vi "Picture to 4bit Picture.vi"() -> ()   [LabVIEW 2014]
uses:
  <userlib>/_OpenG.lib/file/file.llb/Strip Path Extension - Path__ogtk.vi
  <vilib>/Utility/error.llb/Error Cluster From Error Code.vi
  <vilib>/picture/picture.llb/Draw 8-Bit Pixmap.vi
  <vilib>/ErrorRing/Error Ring.xnode
panel:
  in  "Zoom Factor":sgl(slide) scale=0.25..4.0
  out "new picture":picture
  out "Error Out":errorcluster
  in  "Error In":errorcluster
  in  "Path":path=path "C:/Users/mjacobso/Desktop/Draw/Test Images/Test Image.png"
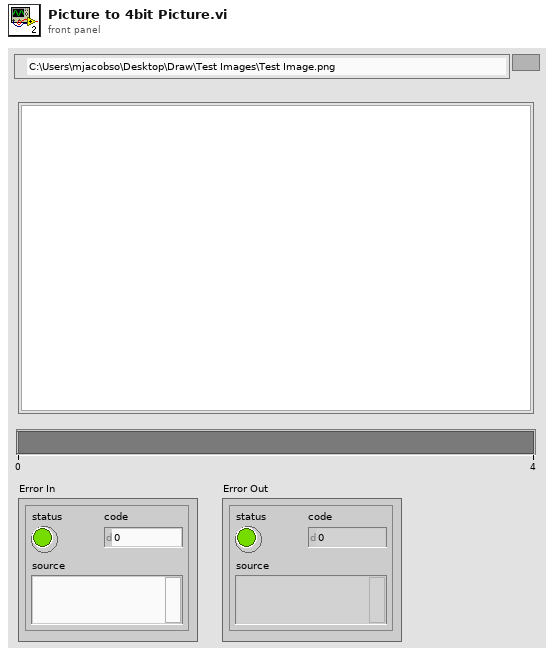
[diagram p1: front panel]
types:
  T1 = typedef "imagedata.ctl" = cluster{"image type":i32, "image depth":i32, "image":u8[], "mask":u8[], "colors":u32[], "Rectangle":cluster{"left":i16, "top":i16, "right":i16, "bottom":i16}}
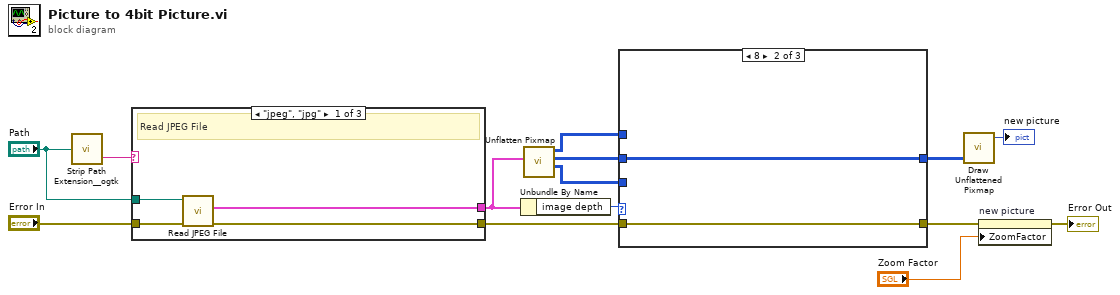
[diagram p0: block diagram]
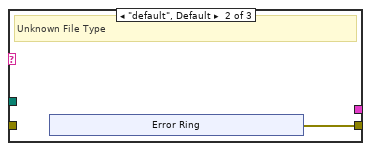
[diagram p4: hidden frame]
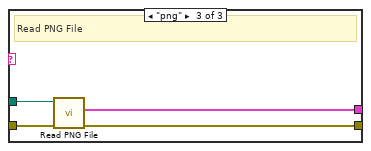
[diagram p5: hidden frame]
diagram:
  n1 = call-poly <userlib>:"Strip Path Extension__ogtk.vi"("path"="Path") -> ("extension"=w14:string)  [unwired: 1 out]
  n2 = case shown="\"jpeg\", \"jpg\"" w14 {
    tunnel: "Path" -> [w18 _ w28]
    tunnel: "Error In" -> [w17 _ w27]
    tunnel: [w16 w19 w25] -> w5
    tunnel: [w15 _ w26] -> w6
    frame "jpeg", "jpg" {
      # "Read JPEG File"
      n3 = call <vilib>:"Read JPEG File.vi"("error in (no error)"=w17, "path to JPEG file"=w18) -> ("error out"=w16:errorcluster, "image data"=w15:T1)  [unwired: 7 in, 1 out]
    }
    frame "default", Default {
      # "Unknown File Type"
      n4 = xnode "Error Ring"() -> ("error out"=w19:errorcluster)
    }
    frame "png" {
      # "Read PNG File"
      n5 = call <vilib>:"Read PNG File.vi"("error in (no error)"=w27, "path to PNG file"=w28) -> ("error out"=w25:errorcluster, "image data"=w26:T1)  [unwired: 7 in, 1 out]
    }
  }
  n6 = Unbundle By Name(w6) -> ("image depth"=w11:i32)
  n7 = call <vilib>:"Unflatten Pixmap.vi"("image data"=w6) -> ("4-bit pixmap"=w10:u8[][], "8-bit pixmap"=w9:u8[][], "24-bit pixmap"=w8:u32[][])  [unwired: 4 in, 4 out]
  n8 = case shown="8" w11 {
    tunnel: w10 -> [_ _ w33]
    tunnel: w9 -> [_ w31 _]
    tunnel: w8 -> [w29 _ _]
    tunnel: w5 -> [w30 w32 w34]
    tunnel: [w30 w32 w34] -> w4
    tunnel: [w29 w31 w33] -> w1
    frame 4 {
    }
    frame 8 {
    }
    frame 24, Default {
    }
  }
  n9 = call-poly <vilib>:"Draw Unflattened Pixmap.vi"("data"=w1) -> ("new picture"=→"new picture":picture)  [unwired: 8 in]
  n10 = property on="new picture" class="Pict"(error in=w4, "ZoomFactor"="Zoom Factor") -> (error out=→"Error Out":errorcluster)  [unwired: 1 in, 1 out]
